vi "ADCP_get_data_packet_details.vi"(0 "ADCP In":refnum<class "ADCP.lvclass">, 5 "NID":u8, 7 "FID":u8, 9 "Data Packet Name":string, 11 "error in (no error)":errorcluster) -> (2 "Parameter names":string[](array[string]), 3 "Node name":string, 4 "ADCP Out":refnum<class "ADCP.lvclass">, 6 "Frame name":string, 8 "Parameters":T3(array[cluster]), 10 "ADCP Data Packet":T2, 15 "error out":errorcluster)   [LabVIEW 2017, in "ADCP.lvclass"]
uses:
  ADCP.lvclass
  ADCP_Data_Packet_Transmit_Mode.ctl
  ADCP.lvclass/ADCP.ctl
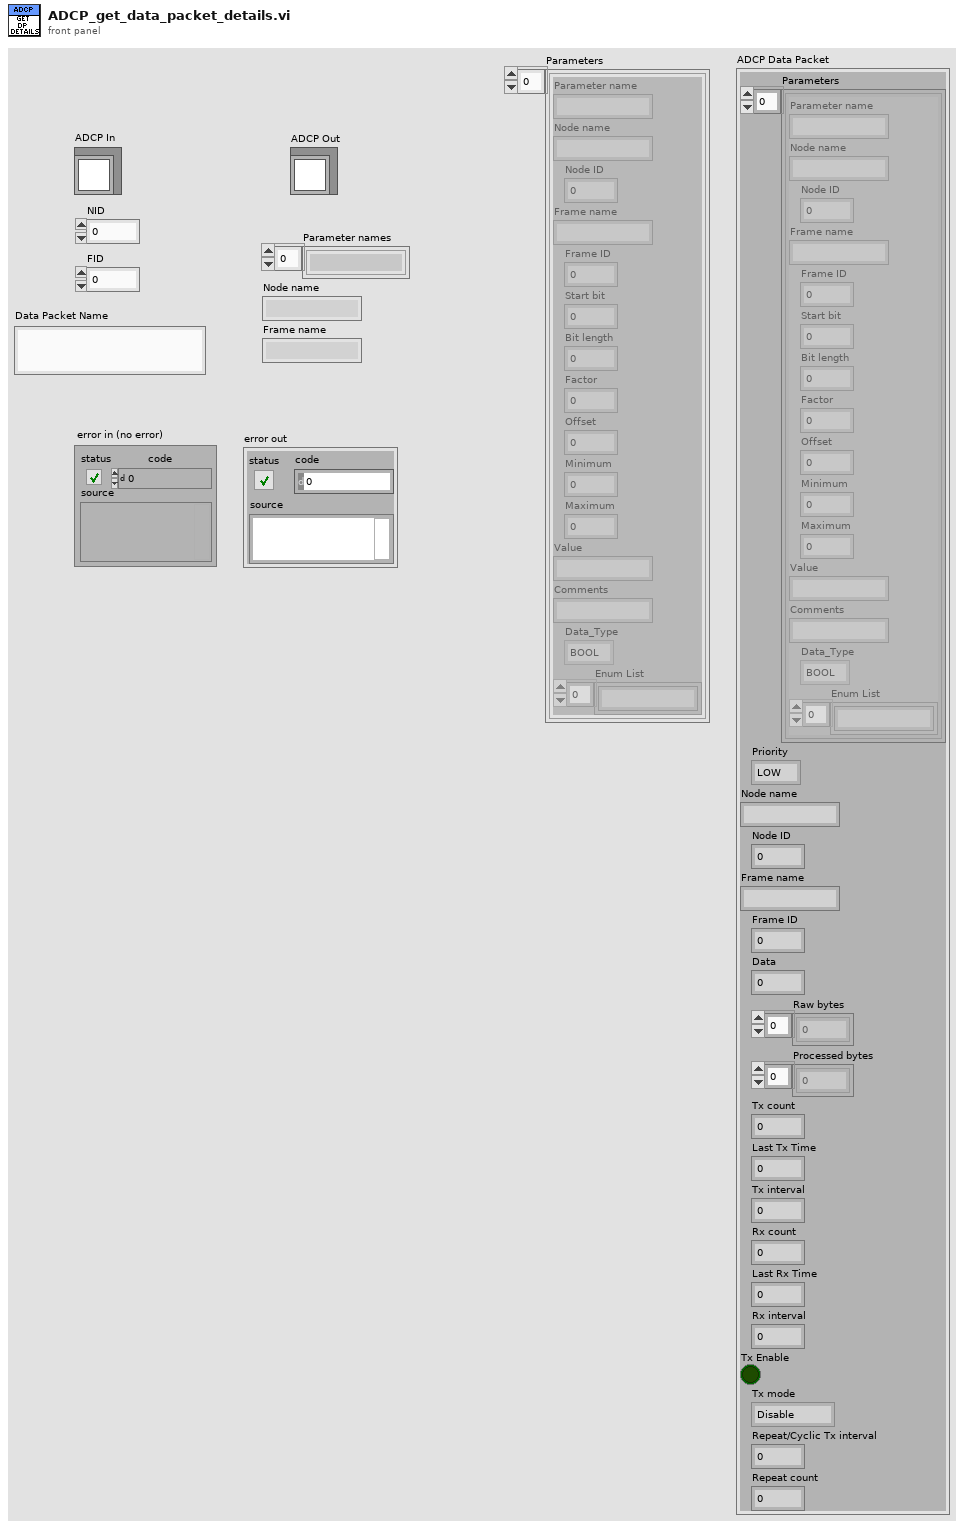
[diagram p1: front panel]
types:
  T1 = typedef "ADCP.lvclass/ADCP_Data_Packet_Transmit_Mode.ctl" = enum16{"Disable", "Single", "Cyclic", "Repeat"}
  T2 = cluster{"Parameters":cluster{"Parameter name":string, "Node name":string, "Node ID":u8, "Frame name":string, "Frame ID":u8, "Start bit":u32, "Bit length":u32, "Factor":dbl, "Offset":dbl, "Minimum":dbl, "Maximum":dbl, "Value":string, "Comments":string, "Data_Type":enum16{"BOOL", "UNSIGNED", "SIGNED", "FLOAT32", "ENUM"}, "Enum List":string[]}[], "Priority":enum16{"LOW", "HIGH"}, "Node name":string, "Node ID":u8, "Frame name":string, "Frame ID":u8, "Data":u32, "Raw bytes":u8[], "Processed bytes":u8[], "Tx count":i32, "Last Tx Time":u32, "Tx interval":u32, "Rx count":i32, "Last Rx Time":u32, "Rx interval":u32, "Tx Enable":bool, "Tx mode":T1, "Repeat/Cyclic Tx interval":u32, "Repeat count":u16}
  T3 = cluster{"Parameter name":string, "Node name":string, "Node ID":u8, "Frame name":string, "Frame ID":u8, "Start bit":u32, "Bit length":u32, "Factor":dbl, "Offset":dbl, "Minimum":dbl, "Maximum":dbl, "Value":string, "Comments":string, "Data_Type":enum16{"BOOL", "UNSIGNED", "SIGNED", "FLOAT32", "ENUM"}, "Enum List":string[]}[]
  T4 = cluster{"Parameters":cluster{"Parameter name":string, "Node name":string, "Node ID":u8, "Frame name":string, "Frame ID":u8, "Start bit":u32, "Bit length":u32, "Factor":dbl, "Offset":dbl, "Minimum":dbl, "Maximum":dbl, "Value":string, "Comments":string, "Data_Type":enum16{"BOOL", "UNSIGNED", "SIGNED", "FLOAT32", "ENUM"}, "Enum List":string[]}[], "Priority":enum16{"LOW", "HIGH"}, "Node name":string, "Node ID":u8, "Frame name":string, "Frame ID":u8, "Data":u32, "Raw bytes":u8[], "Processed bytes":u8[], "Tx count":i32, "Last Tx Time":u32, "Tx interval":u32, "Rx count":i32, "Last Rx Time":u32, "Rx interval":u32, "Tx Enable":bool, "Tx mode":T1, "Repeat/Cyclic Tx interval":u32, "Repeat count":u16}[]
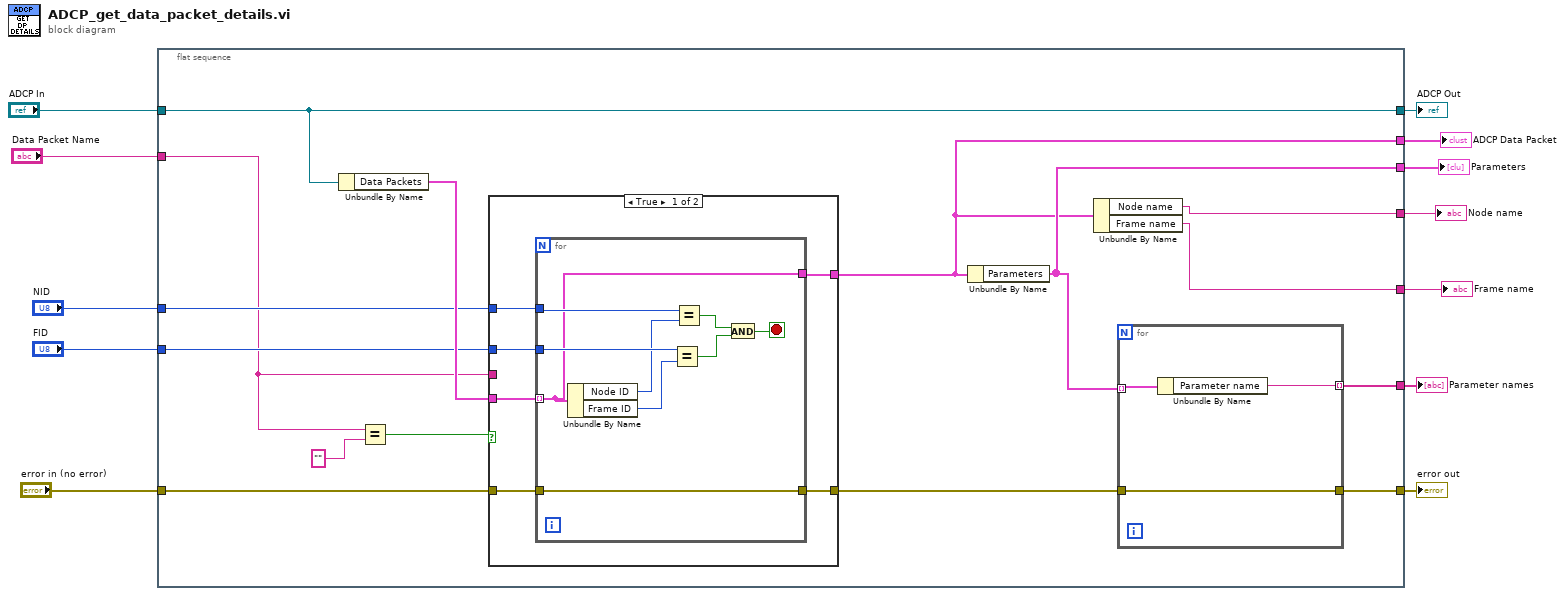
[diagram p0: block diagram]
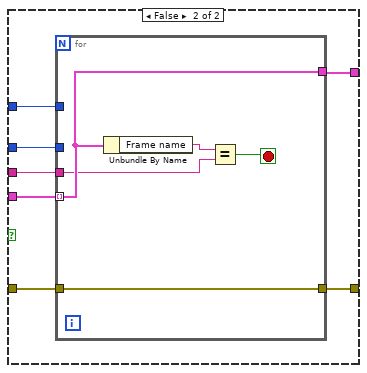
[diagram p2: hidden frame]
diagram:
  n1 = flat-sequence {
    tunnel: "ADCP In" -> [w20]
    tunnel: "error in (no error)" -> [w27]
    tunnel: "NID" -> [w25]
    tunnel: "FID" -> [w24]
    tunnel: [w22] -> w6
    tunnel: [w21] -> w8
    tunnel: [w20] -> w7
    tunnel: [w19] -> w5
    tunnel: [w18] -> w4
    tunnel: [w17] -> w3
    tunnel: [w16] -> w2
    tunnel: "Data Packet Name" -> [w13]
    frame #0 {
      n2 = Unbundle By Name(w20) -> ("Data Packets"=w26:T4)
      n3 = Equal?(x=w13, y="") -> (x = y?=w15:bool)
      n4 = case shown="True" w15 {
        tunnel: w27 -> [w33 w49]
        tunnel: w26 -> [w32 w48]
        tunnel: w25 -> [w31 w47]
        tunnel: w24 -> [w30 w46]
        tunnel: [w29 w45] -> w23
        tunnel: [w28 w44] -> w16
        tunnel: w13 -> [_ w43]
        frame True {
          n5 = for {
            tunnel: w33 -> [w36]
            tunnel: w32 -> [w34] mode=indexing
            tunnel: w31 -> [w42]
            tunnel: w30 -> [w41]
            tunnel: [w36] -> w29
            tunnel: [w34] -> w28
            stop <- w35 stop-if-true
            n6 = Unbundle By Name(w34) -> ("Node ID"=w40:u8, "Frame ID"=w39:u8)
            n7 = Equal?(x=w41, y=w39) -> (x = y?=w37:bool)
            n8 = Equal?(x=w42, y=w40) -> (x = y?=w38:bool)
            n9 = And(x=w38, y=w37) -> (x .and. y?=w35:bool)
          }
        }
        frame False {
          n10 = for {
            tunnel: w49 -> [w54]
            tunnel: w48 -> [w53] mode=indexing
            tunnel: w47 -> [_]
            tunnel: w46 -> [_]
            tunnel: [w54] -> w45
            tunnel: [w53] -> w44
            tunnel: w43 -> [w51]
            stop <- w50 stop-if-true
            n11 = Unbundle By Name(w53) -> ("Frame name"=w52:string)
            n12 = Equal?(x=w52, y=w51) -> (x = y?=w50:bool)
          }
        }
      }
      n13 = Unbundle By Name(w16) -> ("Parameters"=w17:T3)
      n14 = Unbundle By Name(w16) -> ("Node name"=w18:string, "Frame name"=w19:string)
      n15 = for {
        tunnel: w23 -> [w56]
        tunnel: w17 -> [w57] mode=indexing
        tunnel: [w56] -> w22
        tunnel: [w55] -> w21 mode=indexing
        n16 = Unbundle By Name(w57) -> ("Parameter name"=w55:string)
      }
    }
  }
  "Parameter names" <- w8
  "ADCP Out" <- w7
  "error out" <- w6
  "Frame name" <- w5
  "Node name" <- w4
  "Parameters" <- w3
  "ADCP Data Packet" <- w2
